vi "Plotting Data.vi"() -> ()   [LabVIEW 2020]
panel:
  out "GraphPage":refnum<k7>
  out "GraphLayer":refnum<k7>
  out "error out":errorcluster
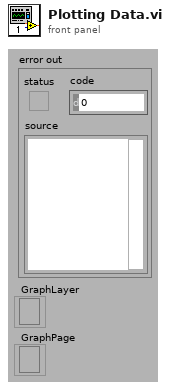
[diagram p1: front panel]
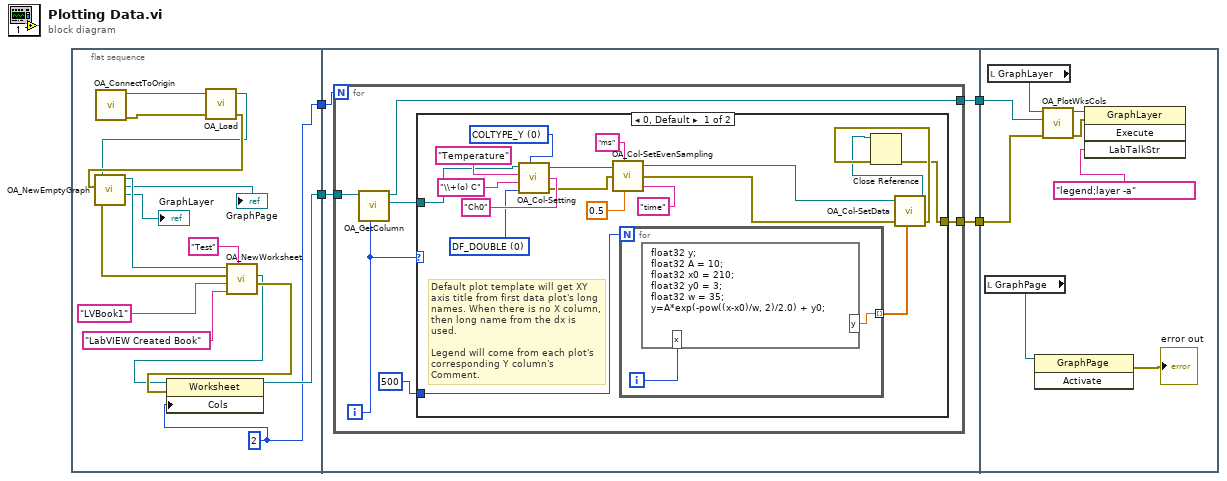
[diagram p0: block diagram]
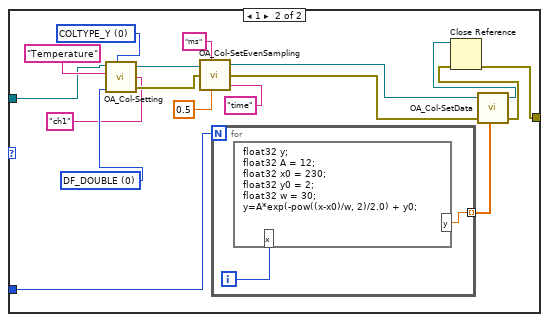
[diagram p2: hidden frame]
diagram:
  n1 = flat-sequence {
    tunnel: [w5] -> w4
    tunnel: [w9] -> w3
    tunnel: w4 -> [w23]
    tunnel: w3 -> [w22]
    tunnel: [w21] -> w2
    tunnel: [w20] -> w1
    tunnel: w2 -> [w75]
    tunnel: w1 -> [w76]
    frame #0 {
      w5 = 2 ("Cols")
      n2 = call "OA_ConnectToOrigin.vi"() -> ("error out"=w10:errorcluster, "Origin.IOApplication"=w13:refnum<k7>)  [unwired: 8 in]
      n3 = call "OA_Load.vi"("error in (no error)"=w10, "Origin.IOApplication"=w13) -> ("error out"=w17:errorcluster, "Origin.IOApplication"=w14:refnum<k7>)  [unwired: 1 in, 1 out]
      n4 = call "OA_NewEmptyGraph.vi"("error in (no error)"=w17, "Origin.IOApplication"=w14) -> ("error out"=w16:errorcluster, "Origin.GraphLayer"=→"GraphLayer":refnum<k7>, "Origin.GraphPage"=→"GraphPage":refnum<k7>, "Origin.IOApplication"=w15:refnum<k7>)  [unwired: 2 in]
      n5 = call "OA_NewWorksheet.vi"("Sheet Name"="Test", "Book LongName"="LabVIEW Created Book", "Book Name"="LVBook1", "error in (no error)"=w16, "Origin.IOApplication"=w15) -> ("error out"=w19:errorcluster, "Origin.Worksheet"=w18:refnum<k7>)  [unwired: 2 in, 1 out]
      n6 = property class="Worksheet"(reference=w18, error in=w19, "Cols"=w5) -> (reference out=w9:refnum<k7>)  [unwired: 1 out]
    }
    frame #1 {
      n7 = for {
        N: w23 -> [_]
        tunnel: w22 -> [w28]
        tunnel: [w27] -> w21
        tunnel: [w26] -> w20
        i -> [w25]
        n8 = call "OA_GetColumn.vi"("Column Name/Index"=w25, "Origin.Worksheet"=w28) -> ("Origin.Column"=w24:refnum<k7>, "Origin.Worksheet"=w26:refnum<k7>)  [unwired: 7 in, 1 out]
        n9 = case shown="0, Default" w25 {
          tunnel: 500 -> [w46 w66]
          tunnel: [w31 w51] -> w27
          tunnel: w24 -> [w34 w53]
          frame 0, Default {
            w38 = 0 items=["DF_NO_CHANGE"=-1, "DF_DOUBLE"=0, "DF_TEXT"=1, "DF_TIME"=2, "DF_DATE"=3, "DF_TEXT_NUMERIC"=9, "DF_FLOAT"=32, "DF_SHORT"=33, "DF_LONG"=34, "DF_CHAR"=35, "DF_BYTE"=38, "DF_USHORT"=39, "DF_ULONG"=40, "DF_COMPLEX"=41] ("DataFormat")
            w42 = 0 items=["COLTYPE_NO_CHANGE"=-1, "COLTYPE_Y"=0, "COLTYPE_NONE"=1, "COLTYPE_ERROR"=2, "COLTYPE_X"=3, "COLTYPE_LABEL"=4, "COLTYPE_Z"=5, "COLTYPE_X_ERROR"=6, "COLTYPE_GROUP"=7, "COLTYPE_SUBJECT"=8] ("Type")
            # "Default plot template will get XY\naxis title from first data plot's long\nnames. When there is no X column, then long name from the dx is used.\n\nLegend will come from each plot's \ncorresponding Y column's Comment."
            n10 = call "OA_Col-Setting.vi"("Origin.Column"=w34, "Type"=w42, "LongName"="Temperature", "Units"="\\+(o) C", "DataFormat"=w38, "Comments"="Ch0") -> ("Origin.Column Out"=w40:refnum<k7>, "error out"=w39:errorcluster)  [unwired: 1 in]
            n11 = call "OA_Col-SetEvenSampling.vi"("Origin.Column"=w40, "Units"="ms", "error in (no error)"=w39, "XInc"=0.5, "LongName"="time") -> ("Origin.Column Out"=w37:refnum<k7>, "error out"=w36:errorcluster)  [unwired: 1 in]
            n12 = for {
              N: w46 -> [_]
              tunnel: [w48] -> w47 mode=indexing
              i -> [w49]
              n13 = formula code="float32 y; \nfloat32 A = 10;\nfloat32 x0 = 210;\nfloat32 y0 = 3;\nfloat32 w = 35;\ny=A*exp(-pow((x-x0)/w, 2)/2.0) + y0;"("x"=w49) -> ("y"=w48:sgl)
            }
            n14 = call "OA_Col-SetData.vi"("Origin.Column"=w37, "error in (no error)"=w36, "data"=w47) -> ("Origin.Column Out"=w30:refnum<k7>, "error out"=w32:errorcluster)  [unwired: 4 in, 1 out]
            n15 = Close Reference(reference=w30, error in (no error)=w32) -> (error out=w31:errorcluster)
          }
          frame 1 {
            w62 = 0 items=["DF_NO_CHANGE"=-1, "DF_DOUBLE"=0, "DF_TEXT"=1, "DF_TIME"=2, "DF_DATE"=3, "DF_TEXT_NUMERIC"=9, "DF_FLOAT"=32, "DF_SHORT"=33, "DF_LONG"=34, "DF_CHAR"=35, "DF_BYTE"=38, "DF_USHORT"=39, "DF_ULONG"=40, "DF_COMPLEX"=41] ("DataFormat")
            w57 = 0 items=["COLTYPE_NO_CHANGE"=-1, "COLTYPE_Y"=0, "COLTYPE_NONE"=1, "COLTYPE_ERROR"=2, "COLTYPE_X"=3, "COLTYPE_LABEL"=4, "COLTYPE_Z"=5, "COLTYPE_X_ERROR"=6, "COLTYPE_GROUP"=7, "COLTYPE_SUBJECT"=8] ("Type")
            n16 = call "OA_Col-Setting.vi"("Origin.Column"=w53, "Type"=w57, "LongName"="Temperature", "DataFormat"=w62, "Comments"="ch1") -> ("Origin.Column Out"=w63:refnum<k7>, "error out"=w64:errorcluster)  [unwired: 2 in]
            n17 = call "OA_Col-SetEvenSampling.vi"("Origin.Column"=w63, "Units"="ms", "error in (no error)"=w64, "XInc"=0.5, "LongName"="time") -> ("Origin.Column Out"=w59:refnum<k7>, "error out"=w58:errorcluster)  [unwired: 1 in]
            n18 = for {
              N: w66 -> [_]
              tunnel: [w67] -> w65 mode=indexing
              i -> [w68]
              n19 = formula code="float32 y; \nfloat32 A = 12;\nfloat32 x0 = 230;\nfloat32 y0 = 2;\nfloat32 w = 30;\ny=A*exp(-pow((x-x0)/w, 2)/2.0) + y0;"("x"=w68) -> ("y"=w67:sgl)
            }
            n20 = call "OA_Col-SetData.vi"("Origin.Column"=w59, "error in (no error)"=w58, "data"=w65) -> ("Origin.Column Out"=w50:refnum<k7>, "error out"=w52:errorcluster)  [unwired: 4 in, 1 out]
            n21 = Close Reference(reference=w50, error in (no error)=w52) -> (error out=w51:errorcluster)
          }
        }
      }
    }
    frame #2 {
      n22 = local read "GraphPage"() -> (w69:refnum<k7>)
      n23 = local read "GraphLayer"() -> (w70:refnum<k7>)
      n24 = invoke class="GraphPage" method="Activate"(reference=w69) -> (error out=→"error out":errorcluster)  [unwired: 2 in, 2 out]
      n25 = call "OA_PlotWksCols.vi"("error in (no error)"=w75, "Origin.Worksheet in"=w76, "Origin.GraphLayer in"=w70) -> ("error out"=w72:errorcluster, "Origin.GraphLayer Out"=w73:refnum<k7>)  [unwired: 5 in, 2 out]
      n26 = invoke class="GraphLayer" method="Execute"(reference=w73, error in=w72, "LabTalkStr"="legend;layer -a") -> ()  [unwired: 1 in, 4 out]
    }
  }
